vi "子VI-读取缺陷测量长宽和面积.vi"(10 "Particle Reports (Pixels)":T1(array[cluster]) {"Orientation" format="%.2f"; "Dimensions"."Height" format="%.2f"; "Dimensions"."Width" format="%.2f"; "Center of Mass"."Y" format="%.2f"; "Center of Mass"."X" format="%.2f"; "Bounding Rect"."Bottom" format="%.2f"; "Bounding Rect"."Right" format="%.2f"; "Bounding Rect"."Top" format="%.2f"; "Bounding Rect"."Left" format="%.2f"; "Number of Holes" format="%.2f"; "Area" format="%.2f"}) -> (2 "测量结果":dbl[][](array[numeric]))   [LabVIEW 2018]
panel:
  out "补几列空数字":dbl[](array[numeric])
  out "高":dbl[](array[numeric])
  out "宽":dbl[](array[numeric])
  out "面积":dbl[](array[numeric])
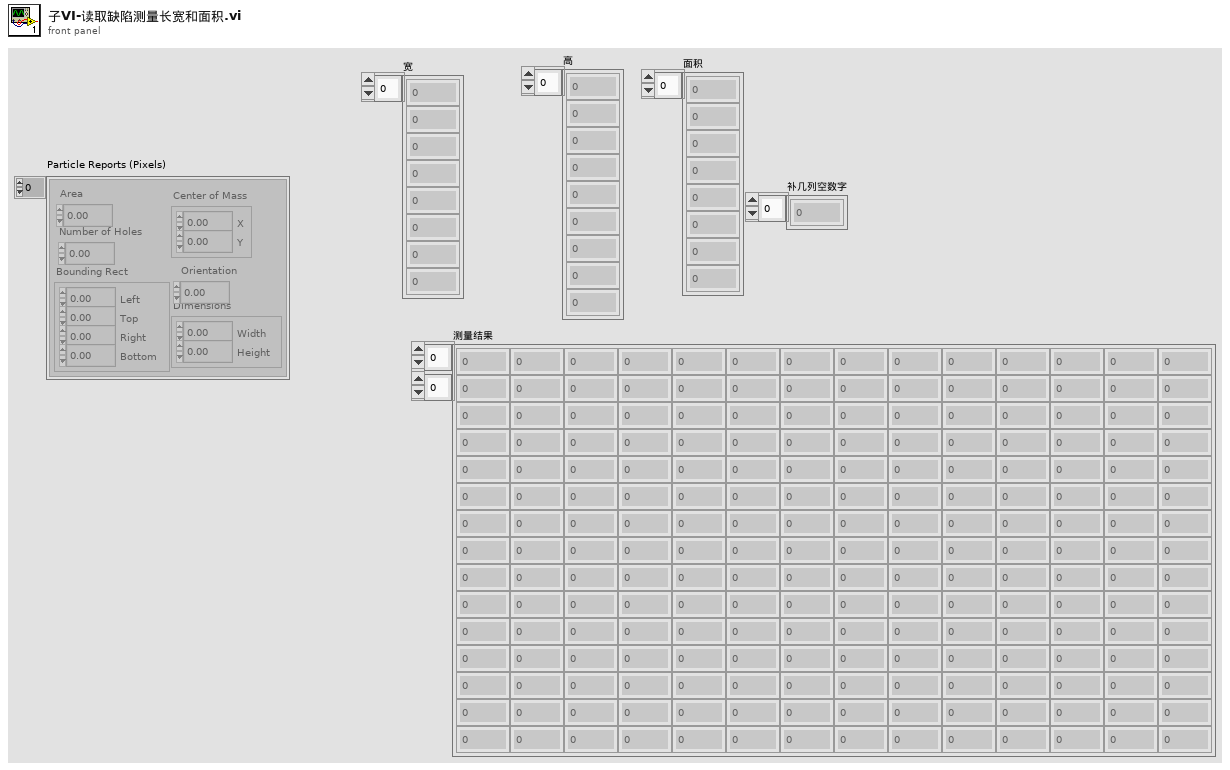
[diagram p1: front panel]
types:
  T1 = cluster{"Area":dbl, "Number of Holes":dbl, "Bounding Rect":cluster{"Left":dbl, "Top":dbl, "Right":dbl, "Bottom":dbl}, "Center of Mass":cluster{"X":dbl, "Y":dbl}, "Orientation":dbl, "Dimensions":cluster{"Width":dbl, "Height":dbl}}[]
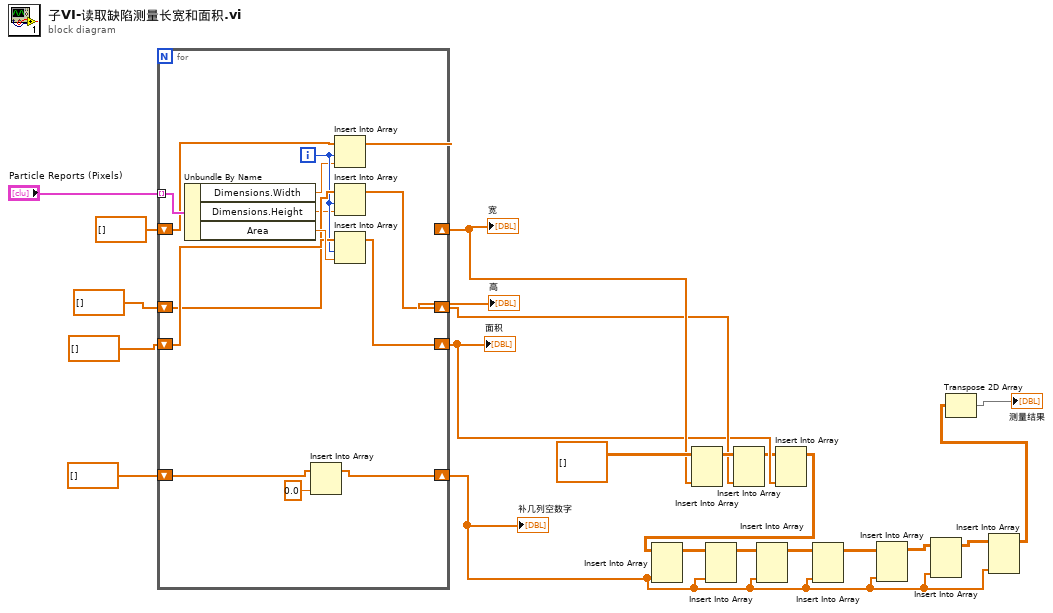
[diagram p0: block diagram]
diagram:
  n1 = for {
    tunnel: "Particle Reports (Pixels)" -> [w35] mode=indexing
    shift-right: [w32] -> w13
    shift-left: dbl[] [] ("数组") -> [w33]
    shift-right: [w27] -> w16
    shift-left: dbl[] [] ("数组") -> [w29]
    shift-right: [w28] -> w14
    shift-left: dbl[] [] ("数组") -> [w31]
    shift-right: [w22] -> w4
    shift-left: dbl[] [] ("数组") -> [w24]
    i -> [w30]
    n2 = Unbundle By Name(w35) -> ("Dimensions.Width"=w25:dbl, "Dimensions.Height"=w26:dbl, "Area"=w34:dbl)
    n3 = Insert Into Array(array=w24, new element=0.0 ("新元素/子数组")) -> (w22:dbl[])  [unwired: 1 in]
    n4 = Insert Into Array(array=w29, index=w30, new element=w25) -> (w27:dbl[])
    n5 = Insert Into Array(array=w31, index=w30, new element=w26) -> (w28:dbl[])
    n6 = Insert Into Array(array=w33, index=w30, new element=w34) -> (w32:dbl[])
  }
  "面积" <- w13
  "宽" <- w16
  "高" <- w14
  "补几列空数字" <- w4
  n7 = Insert Into Array(array=dbl[][] [] ("数组"), new element=w16) -> (w15:dbl[][])  [unwired: 2 in]
  n8 = Insert Into Array(array=w15, new element=w14) -> (w12:dbl[][])  [unwired: 2 in]
  n9 = Insert Into Array(array=w12, new element=w13) -> (w9:dbl[][])  [unwired: 2 in]
  n10 = Insert Into Array(array=w9, new element=w4) -> (w8:dbl[][])  [unwired: 2 in]
  n11 = Insert Into Array(array=w8, new element=w4) -> (w7:dbl[][])  [unwired: 2 in]
  n12 = Insert Into Array(array=w7, new element=w4) -> (w6:dbl[][])  [unwired: 2 in]
  n13 = Insert Into Array(array=w6, new element=w4) -> (w5:dbl[][])  [unwired: 2 in]
  n14 = Insert Into Array(array=w5, new element=w4) -> (w3:dbl[][])  [unwired: 2 in]
  n15 = Insert Into Array(array=w3, new element=w4) -> (w2:dbl[][])  [unwired: 2 in]
  n16 = Insert Into Array(array=w2, new element=w4) -> (w1:dbl[][])  [unwired: 2 in]
  n17 = Transpose 2D Array(2D array=w1) -> (transposed array=→"测量结果":dbl[][])
